vi "getControlDataMPC.vi"(11 "system matricec path":path=path "C:/Users/arnold/Documents/MATLAB/AFM_MPC/data/MPCControls01.csv") -> (1 "AllMatrix":dbl[](array[numeric]), 2 "QP_params":T1={"maxIter"=0, "N"=24, "Ns"=0, "-beta"=-0.9987945556640625, "beta+1"=1.9987945556640625, "SLMAX"=0.039999961853027344, "u0"=0.0400390625}, 3 "ControlParamsMpc":T2={"umax"=3.0, "NS"=0, "ref_f_VEC"=[0.0, 0.0]})   [LabVIEW 2014]
uses:
  <vilib>/Utility/file.llb/Read From Spreadsheet File (DBL).vi
  typeDefs/FXPControlParamsMPC.ctl
  typeDefs/quadProgControls/quadProgParams.ctl
panel:
  # "This vi gets control data from a .csv file. It expects the data in\nthe following format:\n| B,   Ki       |\n| L,    Nbar |\n|K',   Ns      |\n|C',   Nd     |\n|Arn,  ref    |\n|.         0      |\n|.         0      |"
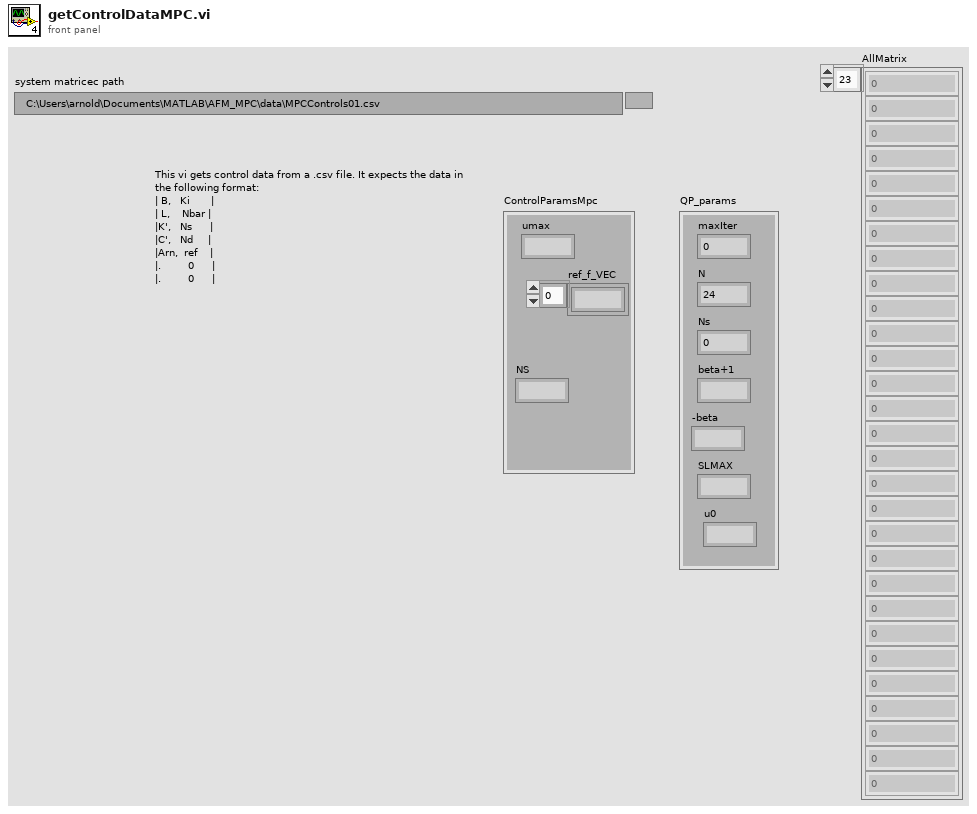
[diagram p1: front panel]
types:
  T1 = typedef "quadProgParams.ctl" = cluster{"maxIter":u16, "N":u16, "Ns":u16, "-beta":fxp<+/-,18,2>, "beta+1":fxp<+/-,18,2>, "SLMAX":fxp<+/-,18,-2>, "u0":fxp<+/-,32,5>}
  T2 = typedef "FXPControlParamsMPC.ctl" = cluster{"umax":fxp<+/-,18,5>, "NS":u8, "ref_f_VEC":fxp<+/-,18,5>[]}
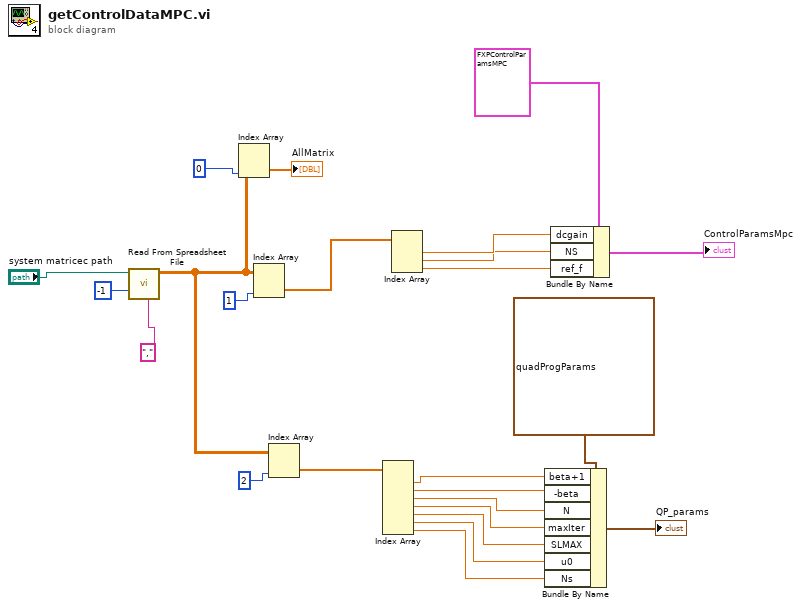
[diagram p0: block diagram]
diagram:
  n1 = call-poly <vilib>:"Read From Spreadsheet File.vi"("delimiter (\\t)"=",", "number of rows (all:-1)"=-1, "file path (dialog if empty)"="system matricec path") -> ("all rows"=w11:dbl[][])  [unwired: 4 in, 4 out]
  n2 = Index Array(array=w11, index (col)=0 ("dimension size")) -> (element=→"AllMatrix":dbl[])  [unwired: 1 in]
  n3 = Index Array(array=w11, index (col)=1 ("dimension size")) -> (element=w23:dbl[])  [unwired: 1 in]
  n4 = Index Array(array=w11, index (col)=2 ("dimension size")) -> (element=w10:dbl[])  [unwired: 1 in]
  n5 = Index Array(array=w10) -> (element #1=w7:dbl, element #2=w6:dbl, element #3=w5:dbl, element #4=w4:dbl, element #5=w3:dbl, element #6=w2:dbl, element #7=w1:dbl)  [unwired: 7 in]
  n6 = Index Array(array=w23) -> (element #1=w15:dbl, element #2=w14:dbl, element #3=w13:dbl)  [unwired: 3 in]
  n7 = Bundle By Name(cluster=T1 {"maxIter"=0, "N"=24, "Ns"=0, "-beta"=-0.9987945556640625, "beta+1"=1.9987945556640625, "SLMAX"=0.039999961853027344, "u0"=0.0400390625} ("QP_params 2"), "beta+1"=w7, "-beta"=w6, "N"=w5, "maxIter"=w4, "SLMAX"=w3, "u0"=w2, "Ns"=w1) -> (→"QP_params":T1)
  n8 = Bundle By Name(cluster=T2 {"umax"=3.0, "NS"=0, "ref_f_VEC"=[0.0, 0.0]} ("ControlParamsMpc 2"), "dcgain"=w15, "NS"=w14, "ref_f"=w13) -> (→"ControlParamsMpc":T2)
